vi "Get Sample Rate.vi"(8 "error in (no error)":errorcluster, 11 "Reference in":T1) -> (0 "error out":errorcluster, 2 "Sample Rate":i32, 3 "Reference out":T1)   [LabVIEW 2016, in "Impulse Data.lvclass"]
uses:
  Impulse Data.lvclass
  Instance handle.ctl
  Impulse Data.lvclass/Impulse Data.ctl
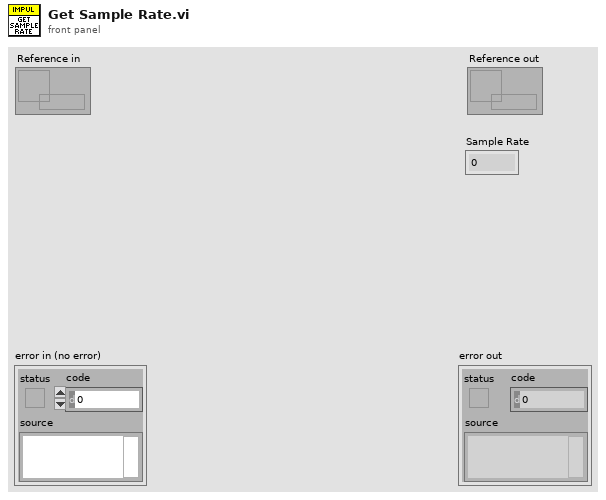
[diagram p1: front panel]
types:
  T1 = typedef "Impulse Data.lvclass/Instance handle.ctl" = refnum<data-value>
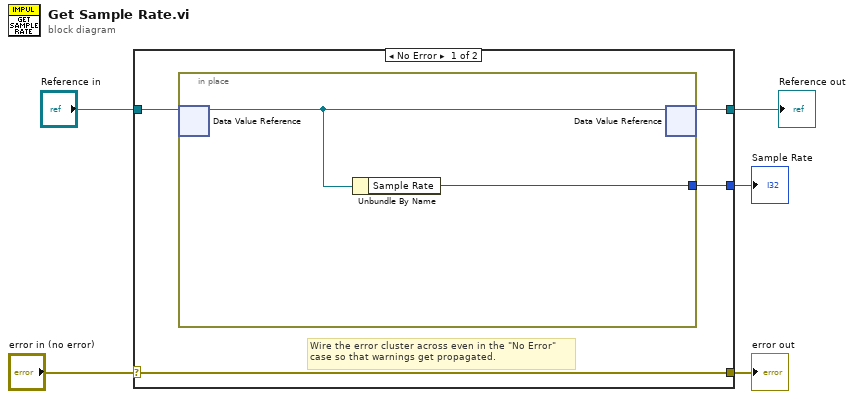
[diagram p0: block diagram]
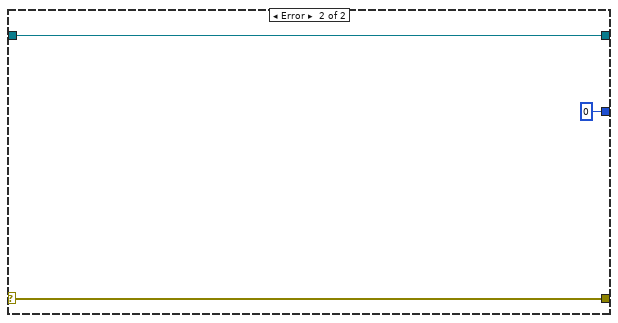
[diagram p2: hidden frame]
diagram:
  n1 = case shown="No Error" "error in (no error)" {
    selector: "error in (no error)" -> [w9 w14]
    tunnel: [w9 w14] -> w4
    tunnel: [w6 0 ("Sample Rate")] -> w3
    tunnel: [w7 w12] -> w2
    tunnel: "Reference in" -> [w8 w12]
    frame No Error {
      # "Wire the error cluster across even in the \"No Error\"\ncase so that warnings get propagated."
      n2 = in-place {
        in-place-border: [w10] -> w6
        n3 = in-place-dvr #1(w8) -> (w11:refnum<class "Impulse Data.lvclass">)  [unwired: 1 out]
        n4 = Unbundle By Name(w11) -> ("Sample Rate"=w10:i32)
        n5 = in-place-dvr #1(w11) -> (w7:T1)  [unwired: 1 out]
      }
    }
    frame Error {
    }
  }
  "error out" <- w4
  "Sample Rate" <- w3
  "Reference out" <- w2
